vi "DataLog Bisection Search LE Start Timestamps.vi"(0 "tag log directory":path, 7 "chunk start timestamps":dbl[](array[numeric]) format="%<%I:%M:%S %p\n%m/%d/%Y>T", 9 "search timestamp":dbl format="%<%I:%M:%S %p\n%m/%d/%Y>T", 11 "error in (no error)":errorcluster) -> (4 "dup tag log directory":path, 8 "dup chunk start timestamps":dbl[](array[numeric]) format="%<%I:%M:%S %p\n%m/%d/%Y>T", 10 "nearest chunk index":i32, 15 "error out":errorcluster)   [LabVIEW 2012]
doc: "Bisection searches an array of chunk start timestamps that must be sorted in increasing order for the last timestamp <= the search timestamp. This operation scales as log(N), where N is the number of timestamps in the array being searched. Some sanity checks are performed so as to ensure that the search always terminates."
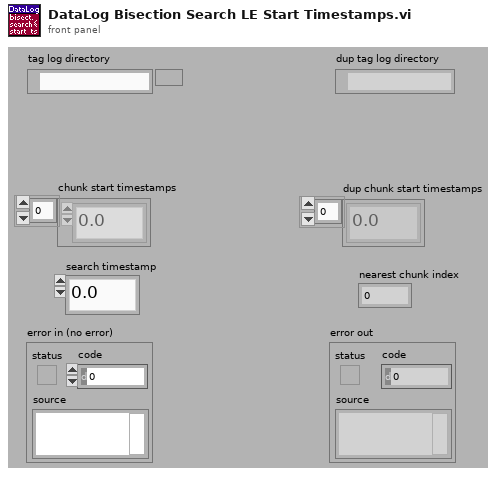
[diagram p1: front panel]
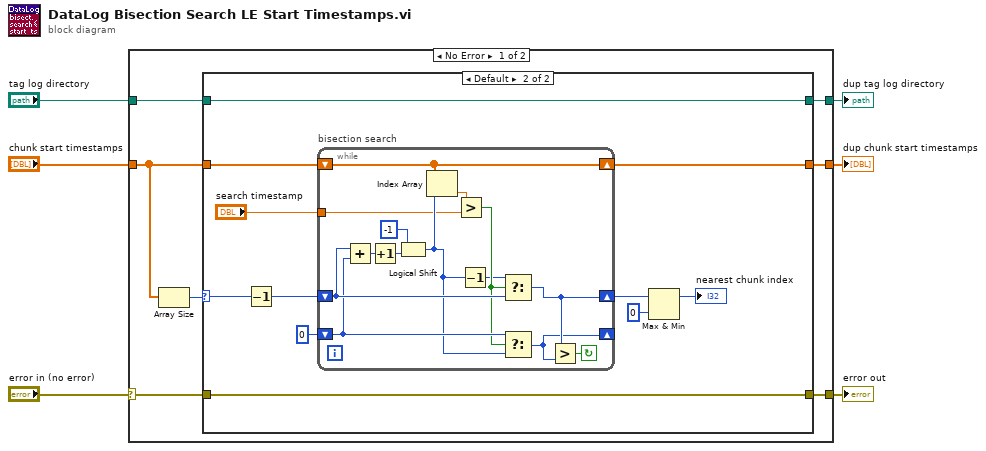
[diagram p0: block diagram]
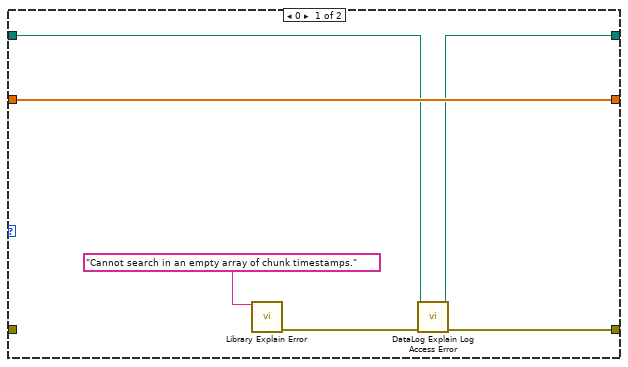
[diagram p2: hidden frame]
diagram:
  n1 = case shown="No Error" "error in (no error)" {
    selector: "error in (no error)" -> [w11 w47]
    tunnel: [w12 w47] -> w6
    tunnel: "tag log directory" -> [w8 w46]
    tunnel: [w7 w46] -> w3
    tunnel: "chunk start timestamps" -> [w10 w45]
    tunnel: [w9 w45] -> w1
    frame No Error {
      n2 = Array Size(array=w10) -> (size(s)=w13:i32)
      n3 = case shown="Default" w13 {
        selector: w13 -> [_ w28]
        tunnel: w10 -> [w18 w30]
        tunnel: [w14 w26] -> w12
        tunnel: w11 -> [_ w26]
        tunnel: [w18 w25] -> w9
        tunnel: w8 -> [w16 w23]
        tunnel: [w15 w23] -> w7
        frame 0 {
          n4 = call "Library Explain Error.vi"("explanation prefix (none)"="Cannot search in an empty array of chunk timestamps." ("explanation")) -> ("explained error"=w17:errorcluster)  [unwired: 14 in]
          n5 = call "DataLog Explain Log Access Error.vi"("tag log directory"=w16, "error in"=w17) -> ("dup tag log directory"=w15:path, "error out"=w14:errorcluster)  [unwired: 12 in]
        }
        frame Default {
          n6 = Decrement(x=w28) -> (x-1=w27:i32)
          n7 = while "bisection search" {
            shift-right: [w36] -> _
            shift-left: 0 -> [w43]
            shift-right: [w42] -> w22
            shift-left: w27 -> [w44]
            tunnel: "search timestamp" -> [w33]
            shift-right: [w31] -> w25
            shift-left: w30 -> [w31]
            stop <- w41 continue-if-true
            n8 = Add(x=w44, y=w43) -> (x+y=w39:i32)
            n9 = Increment(x=w39) -> (x+1=w34:i32)
            n10 = Logical Shift(y=-1, x=w34) -> (x << y=w37:i32)
            n11 = Index Array(array=w31, index=w37) -> (element=w32:dbl)
            n12 = Greater?(x=w32, y=w33) -> (0:w40:bool)
            n13 = Decrement(x=w37) -> (x-1=w35:i32)
            n14 = Select(t=w35, s=w40, f=w44) -> (s? t:f=w42:i32)
            n15 = Select(t=w43, s=w40, f=w37) -> (s? t:f=w36:i32)
            n16 = Greater?(x=w42, y=w36) -> (0:w41:bool)
          }
          n17 = Max & Min(x=w22, y=0) -> (max(x,y)=→"nearest chunk index":i32)  [unwired: 1 out]
        }
      }
    }
    frame Error {
    }
  }
  "error out" <- w6
  "dup tag log directory" <- w3
  "dup chunk start timestamps" <- w1
